vi "MELIII_Lab1.vi"() -> ()   [LabVIEW 2012]
uses:
  <vilib>/express/express shared/transition.llb/Dynamic To Waveform Array.vi
  <vilib>/express/express shared/transition.llb/Waveform Array To Dynamic.vi
  <vilib>/express/express arith-compare/Formula/Block/exnFormulaBlock how many pts in the wave.vi
  <vilib>/express/express shared/ex_Modify Signal Name.vi
  <vilib>/express/express arith-compare/Formula/XNode/ExpressFormulaBlockNode.xnode
panel:
  out "Temperature 4 [K]":dbl
  out "Temperature 3 [K]":dbl
  out "Temperature 2 [K]":dbl
  out "Temperature 1 [K]":dbl
  out "Pressure 2 [MPa]":dbl
  out "Pressure 1 [MPa]":dbl
  out "Pressure vs Time 2":cluster{"Scalar":dbl, "Scalar":dbl}(graph)
  out "Temperature vs Time":T1(graph)
  in  "Atmostpheric \nPressure [psi]":dbl
  in  "Filename":path=path "Z:/adit/Desktop/MEL III/RefrigerationData.lvm"
  in  "Measurement \nPeriod":u32
  in  "?":bool
  # "Still need to fix DAQ input range for P"
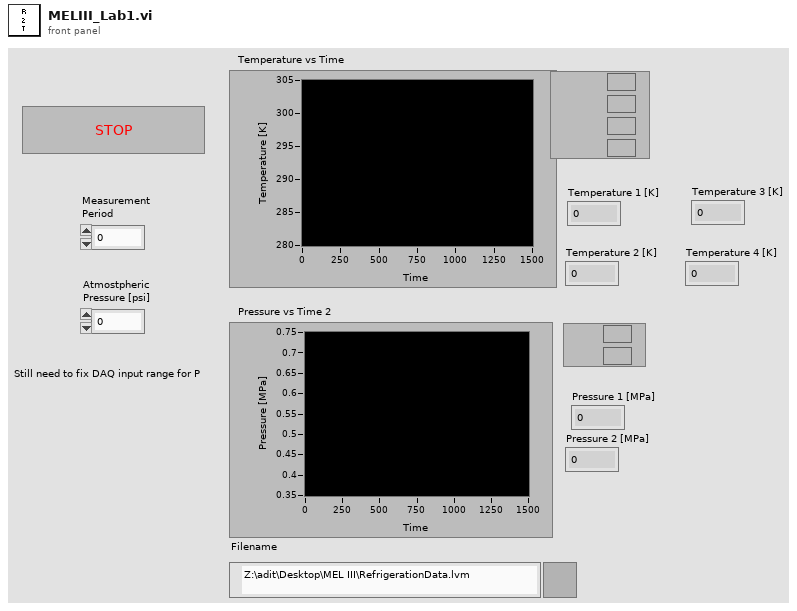
[diagram p1: front panel]
types:
  T1 = cluster{"Result":dbl, "Result":dbl, "Result":dbl, "Result":dbl}
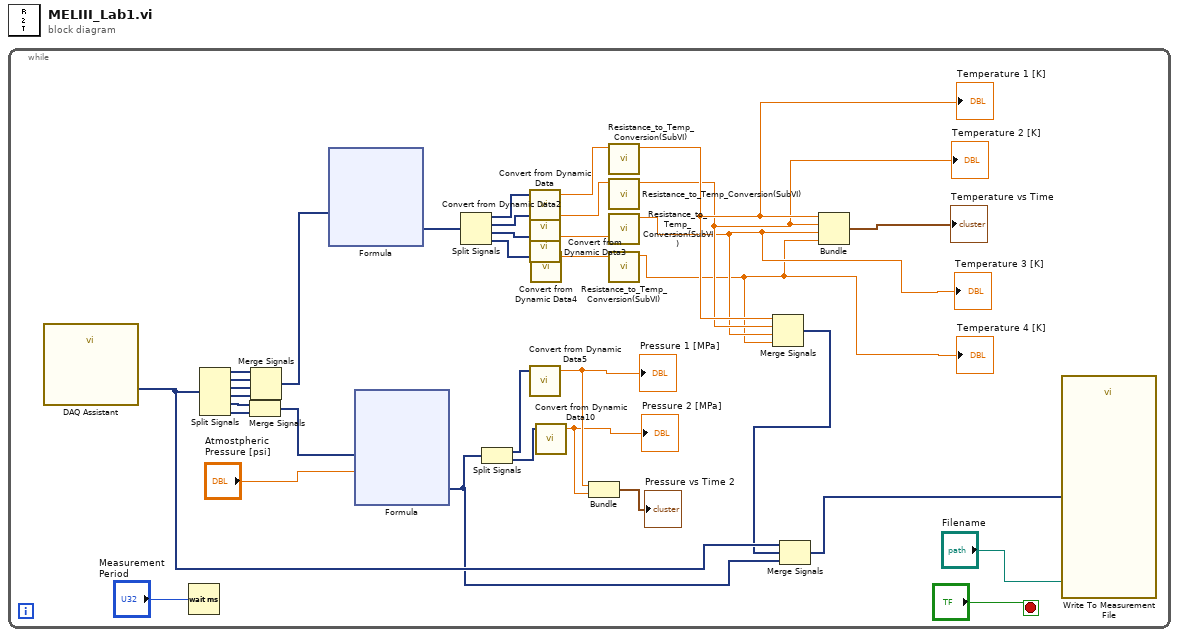
[diagram p0: block diagram]
diagram:
  n1 = while {
    stop <- "?" stop-if-true
    n2 = call "DAQ Assistant"() -> ("data"=w14:dynamicdata)  [unwired: 17 in, 2 out]
    n3 = Wait (ms)(milliseconds to wait="Measurement \nPeriod") -> ()  [unwired: 1 out]
    n4 = Split Signals(w14) -> (w33:dynamicdata, w32:dynamicdata, w31:dynamicdata, w30:dynamicdata, w35:dynamicdata, w34:dynamicdata)  [unwired: 6 in]
    n5 = Merge Signals(w35, w34) -> (w1:dynamicdata)
    n6 = Merge Signals(w33, w32, w31, w30) -> (w29:dynamicdata)
    n7 = xnode "Formula"("V"=w29) -> ("Result"=w27:dynamicdata)  [unwired: 1 in, 1 out]
    n8 = xnode "Formula"("V"=w1, "P_atm"="Atmostpheric \nPressure [psi]") -> ("Result"=w13:dynamicdata)  [unwired: 1 in, 1 out]
    n9 = Split Signals(w27) -> (w26:dynamicdata, w25:dynamicdata, w24:dynamicdata, w23:dynamicdata)  [unwired: 4 in]
    n10 = Split Signals(w13) -> (w12:dynamicdata, w11:dynamicdata)  [unwired: 2 in]
    n11 = call "Convert from Dynamic Data"("Dynamic Data Type"=w26) -> ("Scalar"=w28:dbl)  [unwired: 3 in]
    n12 = call "Convert from Dynamic Data2"("Dynamic Data Type"=w25) -> ("Scalar"=w22:dbl)  [unwired: 3 in]
    n13 = call "Convert from Dynamic Data3"("Dynamic Data Type"=w24) -> ("Scalar"=w21:dbl)  [unwired: 3 in]
    n14 = call "Convert from Dynamic Data5"("Dynamic Data Type"=w12) -> ("Scalar"=w10:dbl)  [unwired: 3 in]
    "Pressure 1 [MPa]" <- w10
    n15 = call "Convert from Dynamic Data4"("Dynamic Data Type"=w23) -> ("Scalar"=w20:dbl)  [unwired: 3 in]
    n16 = call "Convert from Dynamic Data10"("Dynamic Data Type"=w11) -> ("Scalar"=w9:dbl)  [unwired: 3 in]
    "Pressure 2 [MPa]" <- w9
    n17 = Bundle("Scalar"=w10, "Scalar"=w9) -> (→"Pressure vs Time 2":cluster{"Scalar":dbl, "Scalar":dbl})  [unwired: 1 in]
    n18 = call "Resistance_to_Temp_Conversion(SubVI).vi"("Scalar"=w28) -> ("Result"=w5:dbl)  [unwired: 10 in]
    "Temperature 1 [K]" <- w5
    n19 = call "Resistance_to_Temp_Conversion(SubVI).vi"("Scalar"=w22) -> ("Result"=w4:dbl)  [unwired: 10 in]
    "Temperature 2 [K]" <- w4
    n20 = call "Resistance_to_Temp_Conversion(SubVI).vi"("Scalar"=w21) -> ("Result"=w3:dbl)  [unwired: 10 in]
    "Temperature 3 [K]" <- w3
    n21 = call "Resistance_to_Temp_Conversion(SubVI).vi"("Scalar"=w20) -> ("Result"=w2:dbl)  [unwired: 10 in]
    "Temperature 4 [K]" <- w2
    n22 = Merge Signals(w5, w4, w3, w2) -> (w6:dynamicdata)
    n23 = Merge Signals(w14, w6, w13) -> (w19:dynamicdata)
    n24 = Bundle("Result"=w5, "Result"=w4, "Result"=w3, "Result"=w2) -> (→"Temperature vs Time":T1)  [unwired: 1 in]
    n25 = call "Write To Measurement File"("Signals"=w19, "Filename"="Filename") -> ()  [unwired: 15 in, 3 out]
  }
